vi "CAN Write.vi"(10 "MessageBuffer":T1, 11 "Channel":u16) -> (2 "MessageBuffer out":T1, 3 "function return":u32)   [LabVIEW 2020, in "PCANBasic.lvlib"]
doc: "TPCANStatus __stdcall CAN_Write(\n TPCANHandle Channel, \n TPCANMsg* MessageBuffer);"
uses:
  PCANBasic.lvlib
  <userlib>/PCANBasic/PCANBasic.dll
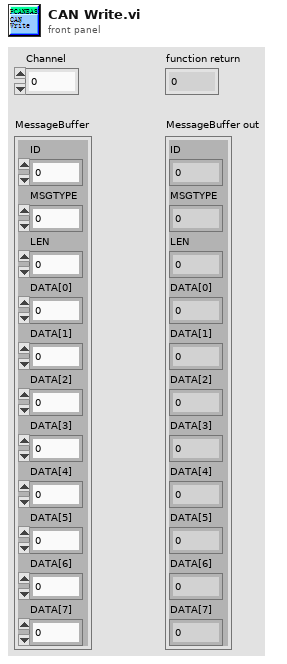
[diagram p1: front panel]
types:
  T1 = cluster{"ID":u32, "MSGTYPE":u8, "LEN":u8, "DATA[0]":u8, "DATA[1]":u8, "DATA[2]":u8, "DATA[3]":u8, "DATA[4]":u8, "DATA[5]":u8, "DATA[6]":u8, "DATA[7]":u8}
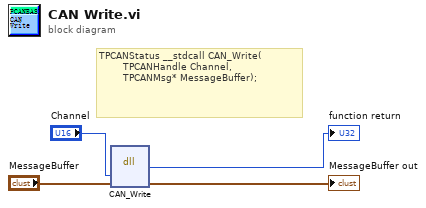
[diagram p0: block diagram]
diagram:
  # "TPCANStatus __stdcall CAN_Write(\n        TPCANHandle Channel, \n        TPCANMsg* MessageBuffer);"
  n1 = dll-call lib="D:/Program Files (x86)/National Instruments/LabVIEW 2020/user.lib/PCANBasic/PCANBasic.*" fn="CAN_Write"("Channel"="Channel", "MessageBuffer"="MessageBuffer") -> (→"function return":u32, "MessageBuffer"=→"MessageBuffer out":T1)  [unwired: 4 in, 2 out]
